vi "svx_Orbit Event Scale Read.vi"(4 "error in (no error)":errorcluster, 6 "Container State":T2, 7 "Display State In":T1) -> (0 "error out":errorcluster, 2 "Value":refnum<user-event>, 3 "Display State Out":T1)   [LabVIEW 2017, in "SVX Orbit.xctl"]
uses:
  <vilib>/addons/_XControls/Orbit Plot/SVX Orbit.xctl
  <vilib>/_xctls/Container State.ctl
  <vilib>/addons/_XControls/Orbit Plot/subVIs/svx_Orbit State.ctl
  <vilib>/addons/_XControls/Orbit Plot/subVIs/svx_Orbit Internal State.ctl
  <vilib>/addons/_XControls/Orbit Plot/subVIs/svx_Orbit Bounds.ctl
  <vilib>/_xctls/XControlSupport.lvlib
panel:
  # "Replace the Value Indicator below with an Indicator of desired type.\nDo not remove this Indicator or the others from the connector pane. \nDo not change the connector pane pattern.\nThe Value Indicator should always be the second terminal from top on the output side in the connector pane."
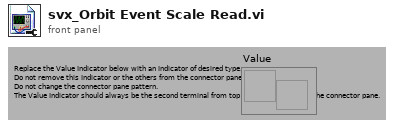
[diagram p1: front panel]
types:
  T1 = typedef "SVX Orbit.xctl/svx_Orbit State.ctl" = cluster{"State Queue":refnum<queue>, "Old State":variant}
  T2 = typedef "XControlSupport.lvlib/Container State.ctl" = cluster{"Indicator?":bool, "Run Mode?":bool, " Refnum":refnum<vi>}
  T3 = typedef "SVX Orbit.xctl/svx_Orbit Internal State.ctl" = cluster{"X Scale":cluster{"Name":string, "FString":string, "Major Color":u32, "Minor Color":u32, "Scale Visible":bool, " Label Visible":bool, "Grid Style":u16}, "Y Scale":cluster{"Name":string, "FString":string, "Major Color":u32, "Minor Color":u32, "Scale Visible":bool, " Label Visible":bool, "Grid Style":u16}, "Plot":cluster{"Point Style":u8, "Line Width":u8, "Line Style":u8, "Plot Color":u32, "Point/fill":u32}, "Arrow/Crosshair Color":u32, "Tacho Point Color":u32, "Container Bounds":T4, "Axis Maximum":dbl, "Probe Angles":cluster{"Angle X":dbl, "Angle Y":dbl}, "Background Color":u32, "Cursor":cluster{"Cursor Point Style":u8, "Cursor Style":u8, "Cursor Line Width":u8, "Cursor Line Style":u8, "Cursor Color":u32, "Cursor Name Visible":bool, "Cursor Visible":bool, "Cursor Position":cluster{"X":dbl, "Y":dbl}, "Cursor Index":i32, "Cursor Lock":bool}, "Elliptical Info":cluster{"a":dbl, "b":dbl, "e":dbl, "ang":dbl}[], "Legend Visible":bool, "Scale Range Change":refnum<user-event>, "Strings[]":cluster{"Custom pair name":bool, "Row Strings []":string[], "Column Strings []":string[]}, "Index":cluster{"pair index":i32, "order index":i32}[], " Parents Tags":string[], "Children Tags":string[], "Open?":bool[], "Label":string, "Legend Width":u32, "Pair Strings Changed?":bool, "Size":i32[], "Legend Background":u32, "Legend Font":u32, "Cursor Release":refnum<user-event>, "Autoscale":bool, "Precession Direction":enum16{"forward", "backward"}[], "Item Width":u32, "User Pair Strings []":string[], "Users Order Strings []":string[], "Autoscale Once":bool, "Property Write":refnum<queue>}
  T4 = typedef "SVX Orbit.xctl/svx_Orbit Bounds.ctl" = cluster{"Width":u32, "Height":u32}
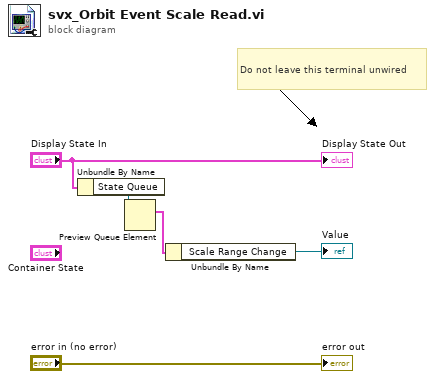
[diagram p0: block diagram]
diagram:
  # "Do not leave this terminal unwired"
  n1 = Unbundle By Name("Display State In") -> ("State Queue"=w3:refnum<queue>)
  n2 = Preview Queue Element(queue=w3) -> (element=w2:T3)  [unwired: 2 in, 3 out]
  n3 = Unbundle By Name(w2) -> ("Scale Range Change"=→"Value":refnum<user-event>)
  "error out" <- "error in (no error)"
  "Display State Out" <- "Display State In"
